vi "Elevator Immediate.vi"(7 "Description":string, 8 "Command Info In":T1, 9 "Setpoint Pinch":dbl, 10 "Deadband Value":dbl=0.05, 11 "Setpoint":dbl) -> (0 "Command Info Out":T1)   [LabVIEW 2017]
doc: "This template is useful for immediate subsystem actions that do not need deadband filtering\n\nBe sure to right-click and select New from Template and save with a new command name."
uses:
  <vilib>/Rock Robotics/WPI/Framework/Command Status Info.ctl
  <vilib>/Rock Robotics/WPI/Framework/Completion Status.ctl
  <vilib>/Rock Robotics/WPI/Framework/Completion Notifier.ctl
  Implementation/Elevator Setpoints.ctl
  Implementation/Elevator Operations.ctl
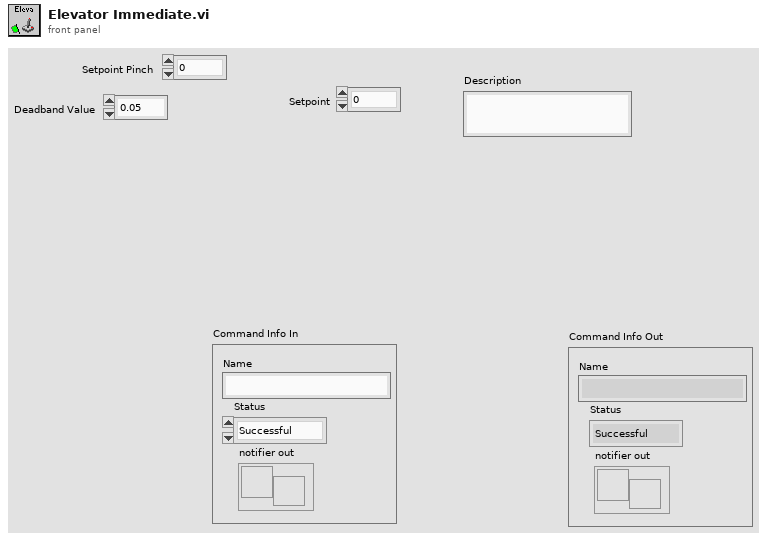
[diagram p1: front panel]
types:
  T1 = typedef "Command Status Info.ctl" = cluster{"Name":string, "Status":T2, "notifier out":T3}
  T2 = typedef "Completion Status.ctl" = enum16{"Successful", "Aborted", "Incomplete"}
  T3 = typedef "Completion Notifier.ctl" = refnum<notifier>
  T4 = typedef "Elevator Setpoints.ctl" = cluster{"Operation":T5, "Setpoint":dbl, "Duration":dbl}
  T5 = typedef "Elevator Operations.ctl" = enum16{"Reserve", "Read Current", "Immediate", "Go to Height", "Fudge Up", "Fudge Down", "Zero Elevator Encoders", "Go to A", "Hold A", "Hold A for Duration"}
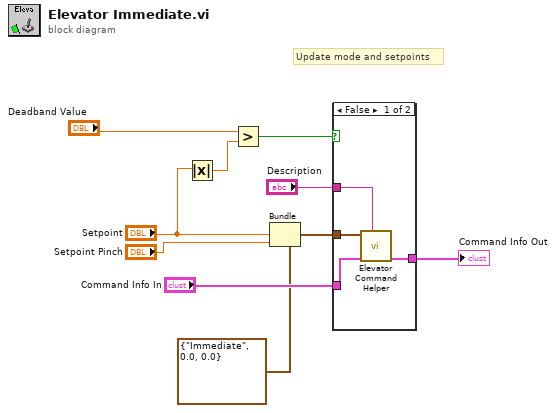
[diagram p0: block diagram]
diagram:
  # "Update mode and setpoints"
  n1 = Absolute Value(x="Setpoint") -> (abs(x)=w4:dbl)
  n2 = Greater?(x="Deadband Value", y=w4) -> (0:w3:bool)
  n3 = Bundle(cluster=T4 {"Operation"=enum."Immediate", "Setpoint"=0.0, "Duration"=0.0} ("SubSystem Data"), "Setpoint"="Setpoint", "Duration"="Setpoint Pinch") -> (w6:T4)  [unwired: 1 in]
  n4 = case shown="False" w3 {
    tunnel: [w14 w15] -> w10
    tunnel: "Command Info In" -> [w13 w15]
    tunnel: "Description" -> [w12 _]
    tunnel: w6 -> [w11 _]
    frame False {
      n5 = call "Elevator Command Helper.vi"("Description"=w12, "Command Info In"=w13, "SubSystem Data"=w11) -> ("Command Info Out"=w14:T1)  [unwired: 6 in, 2 out]
    }
    frame True {
    }
  }
  "Command Info Out" <- w10
